vi "NI App Web Server.vi"() -> ()   [LabVIEW 2023]
uses:
  <vilib>/httpClient/POSTBuffer.vi
  Bad Idea Globals.vi
  <vilib>/httpClient/LabVIEWHTTPClient.lvlib
  <vilib>/Utility/TDMS File Viewer/NI_TDMS File Viewer.lvlib
panel:
  in  "Shutdown":bool
  in  "Freq":dbl=8.0
  in  "Phase":dbl
  in  "Amplitude":dbl=2.0
  out "Latest":waveform(dbl)(graph) caption="Latest Waveform from WebService"
  in  "Save":bool
  in  "Live":bool
  in  "Stop":bool
  in  "Start":bool
  out "WS_Shutdown":bool
  out "Running?":bool
  out "Commands":string[](array[string])
  out "Live":dynamicdata(graph) caption="Live Waveform (generated while \"Running\")"
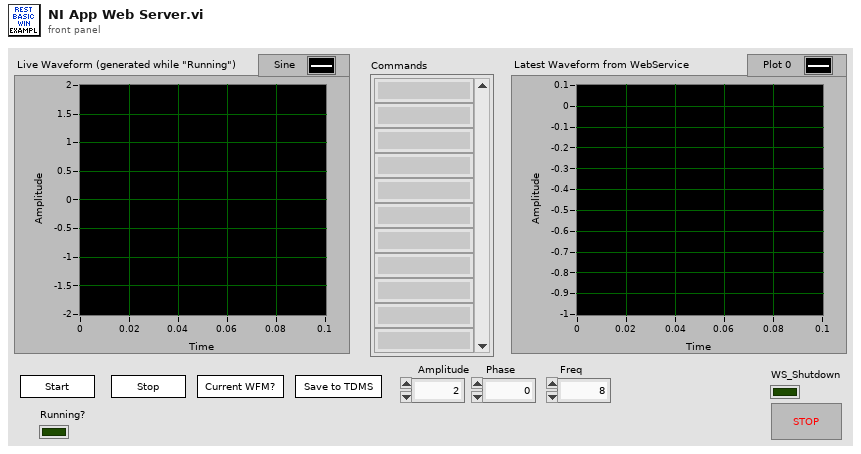
[diagram p1: front panel]
types:
  T1 = cluster{"Running":bool, "Amplitude":dbl, "Phase":dbl, "Freq":dbl}
  T2 = typedef "LabVIEWHTTPClient.lvlib/ClientHandle.ctl" = refnum<k1>
  T3 = enum16{"open", "open or create", "create or replace", "create", "open (read-only)"}
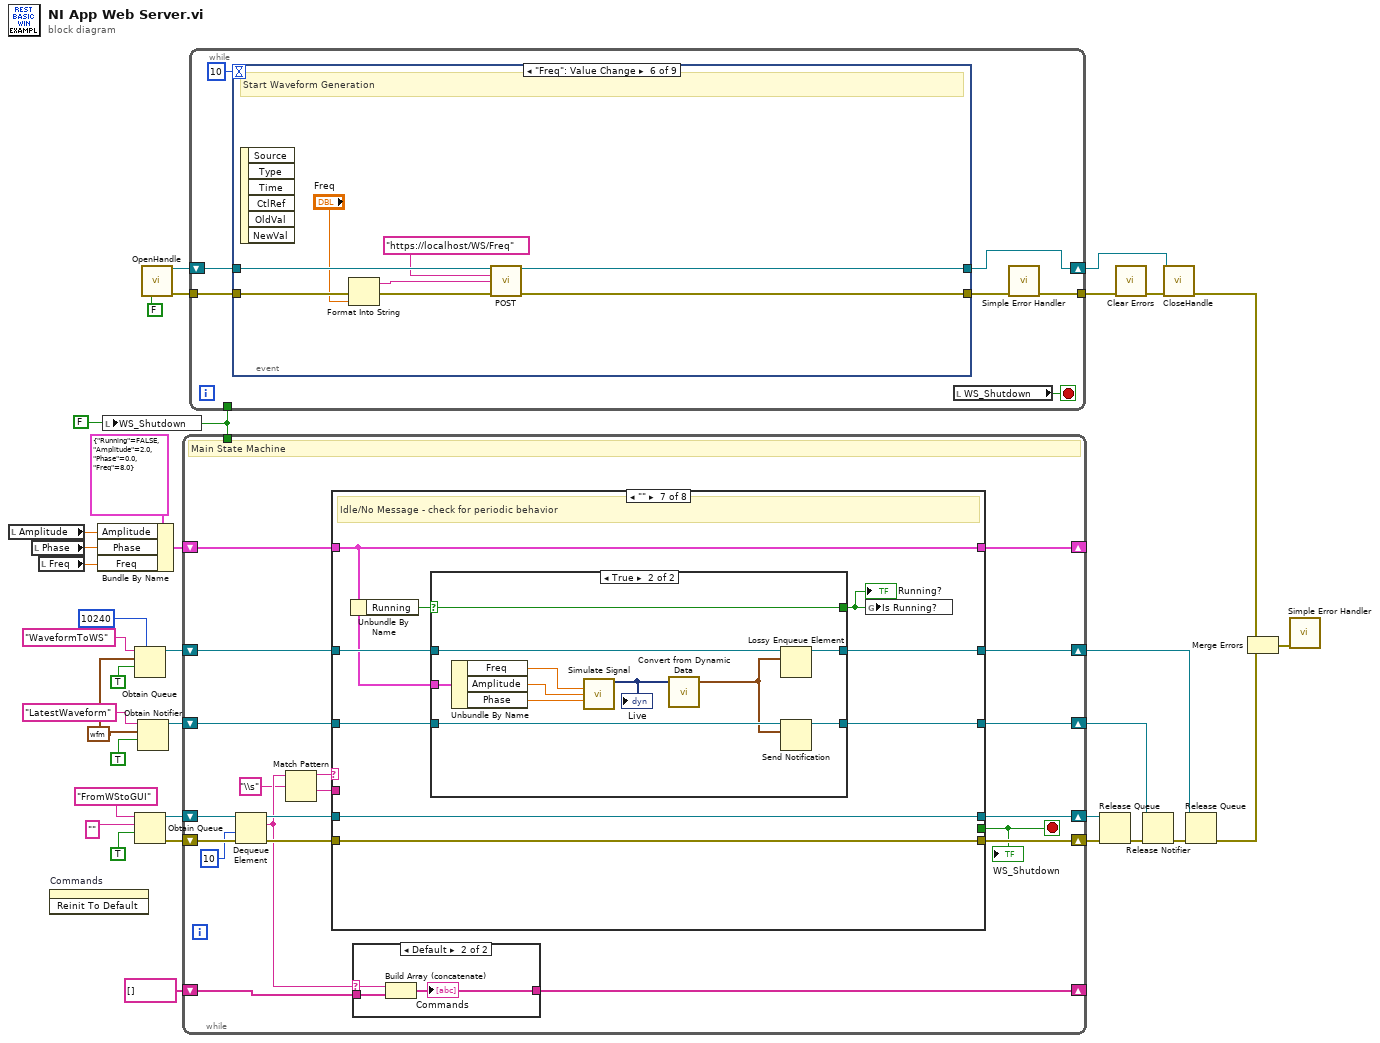
[diagram p0: block diagram]
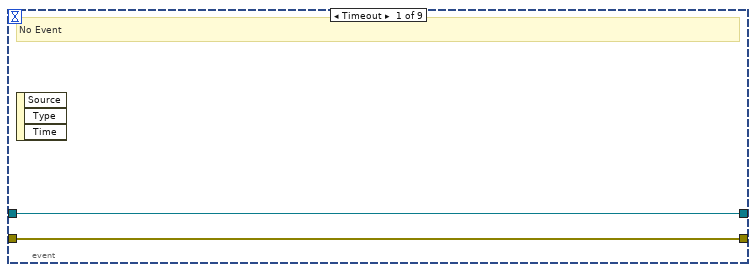
[diagram p2: hidden frame]
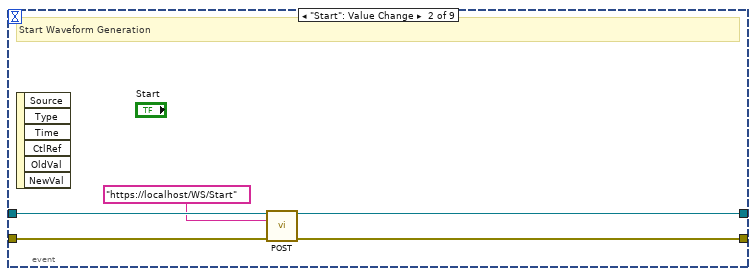
[diagram p3: hidden frame]
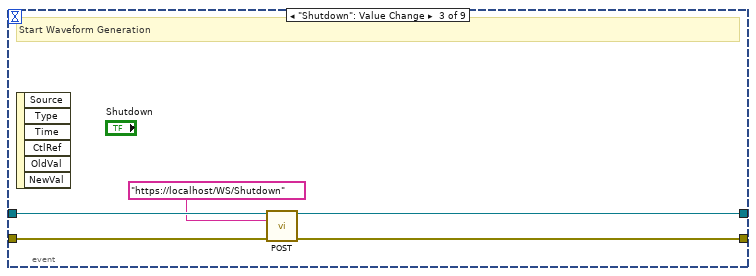
[diagram p4: hidden frame]
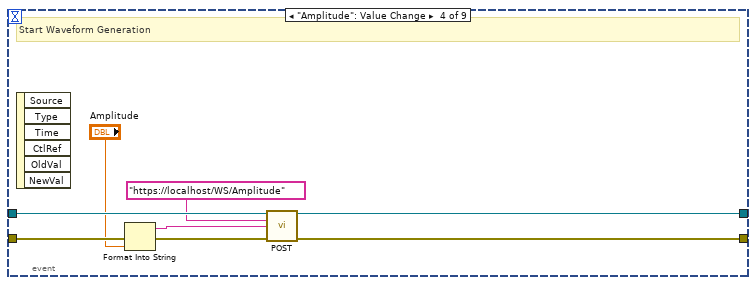
[diagram p5: hidden frame]
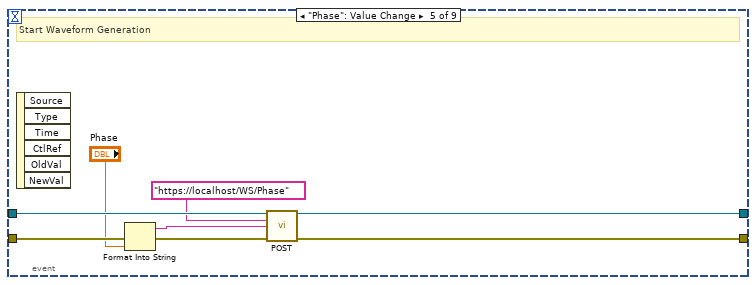
[diagram p6: hidden frame]
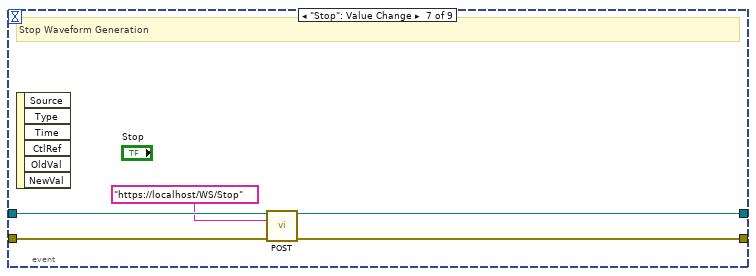
[diagram p7: hidden frame]
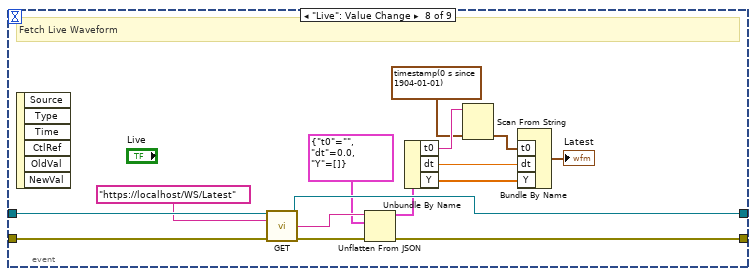
[diagram p8: hidden frame]
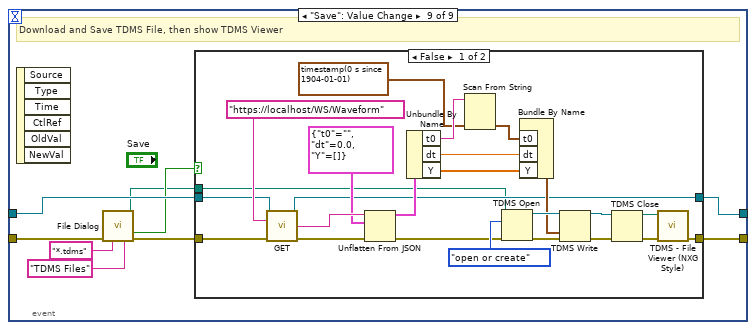
[diagram p9: hidden frame]
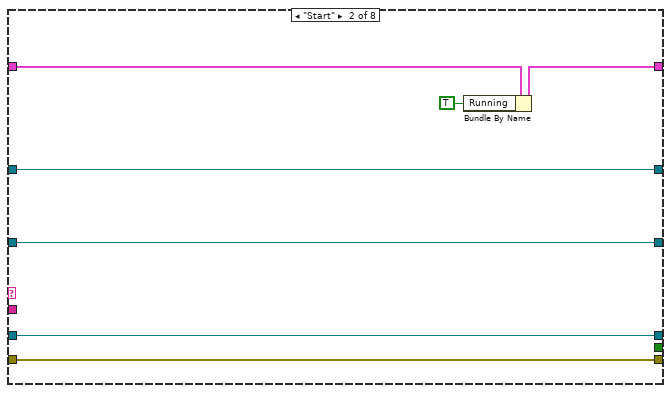
[diagram p13: hidden frame]
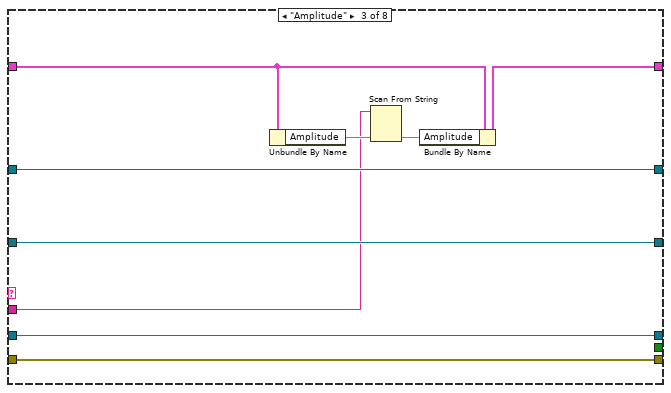
[diagram p14: hidden frame]
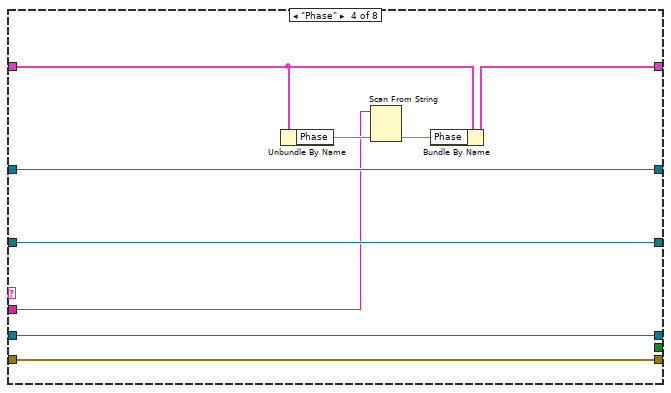
[diagram p15: hidden frame]
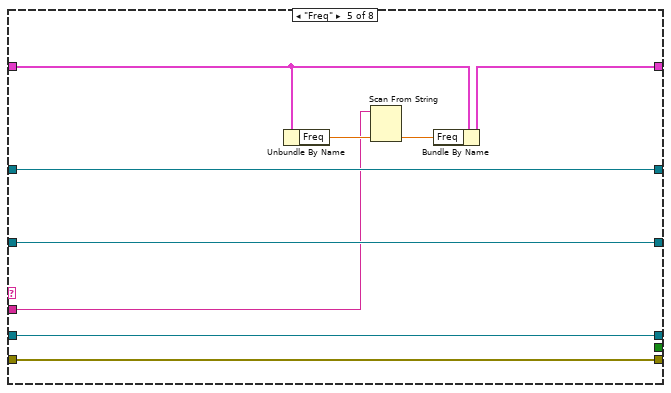
[diagram p16: hidden frame]
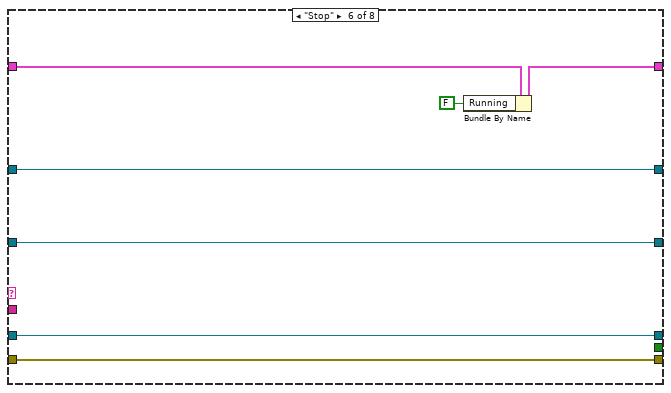
[diagram p17: hidden frame]
diagram:
  w15 = FALSE
  w28 = waveform(dbl) {"t0"=timestamp(0 s since 1904-01-01), "dt"=1.0, "Y"=[]}
  n1 = local read "Amplitude"() -> (w3:dbl)
  n2 = local read "Phase"() -> (w2:dbl)
  n3 = local read "Freq"() -> (w1:dbl)
  n4 = invoke on="Commands" class="Arr (strict)" method="Reinit To Default"() -> ()  [unwired: 3 in, 3 out]
  n5 = Bundle By Name(cluster=T1 {"Running"=FALSE, "Amplitude"=2.0, "Phase"=0.0, "Freq"=8.0}, "Amplitude"=w3, "Phase"=w2, "Freq"=w1) -> (w5:T1)
  n6 = local write "WS_Shutdown"(w15) -> ()
  n7 = Obtain Queue(max queue size (-1, unlimited)=10240, name (unnamed)="WaveformToWS", element data type=w28, create if not found? (T)=TRUE) -> (queue out=w27:refnum<queue>)  [unwired: 1 in, 2 out]
  n8 = Obtain Queue(name (unnamed)="FromWStoGUI", element data type="", create if not found? (T)=TRUE) -> (queue out=w32:refnum<queue>, error out=w33:errorcluster)  [unwired: 2 in, 1 out]
  n9 = Obtain Notifier(name (unnamed)="LatestWaveform", notification data type=w28, create if not found? (T)=TRUE) -> (notifier out=w29:refnum<notifier>)  [unwired: 1 in, 2 out]
  n10 = call <vilib>:"OpenHandle.vi"("verify server(true)"=FALSE) -> ("client handle out"=w19:T2, "error out"=w18:errorcluster)  [unwired: 13 in]
  n11 = while "Send to RT" {
    shift-right: [w49] -> w30
    shift-left: w33 -> [w55]
    shift-right: [w50] -> w31
    shift-left: w32 -> [w54]
    shift-right: [w47] -> w24
    shift-left: w29 -> [w48]
    shift-right: [w45] -> w23
    shift-left: w27 -> [w46]
    shift-right: [w43] -> _
    shift-left: w5 -> [w44]
    shift-right: [w41] -> _
    shift-left: string[] [] -> [w42]
    tunnel: w15 -> [_]
    stop <- w36 stop-if-true
    # "Main State Machine"
    n12 = Dequeue Element(queue=w54, timeout in ms (-1)=10, error in (no error)=w55) -> (queue out=w51:refnum<queue>, element=w40:string, error out=w52:errorcluster)  [unwired: 1 out]
    n13 = Match Pattern(string=w40, regular expression="\\s") -> (before substring=w39:string, after substring=w37:string)  [unwired: 1 in, 2 out]
    n14 = case shown="\"\"" w39 {
      tunnel: w52 -> [w63 w70 w79 w88 w97 w104 w113 w133]
      tunnel: w51 -> [w64 w71 w80 w89 w98 w105 w114 w134]
      tunnel: [w64 w71 w80 w89 w98 w105 w114 w134] -> w50
      tunnel: [w63 w70 w79 w88 w97 w104 w113 w133] -> w49
      tunnel: [_ _ _ _ _ _ _ TRUE] -> w36
      tunnel: w48 -> [w62 w69 w78 w87 w96 w103 w110 w131]
      tunnel: [w62 w69 w78 w87 w96 w103 w108 w131] -> w47
      tunnel: w46 -> [w61 w68 w77 w86 w95 w102 w111 w130]
      tunnel: [w61 w68 w77 w86 w95 w102 w109 w130] -> w45
      tunnel: w44 -> [w60 w65 w74 w83 w92 w99 w107 w129]
      tunnel: [w60 w66 w76 w85 w94 w100 w107 w129] -> w43
      tunnel: w37 -> [_ _ w72 w81 w90 _ _ _]
      frame Default {
      }
      frame "Start" {
        n15 = Bundle By Name(cluster=w65, "Running"=TRUE) -> (w66:T1)
      }
      frame "Amplitude" {
        n16 = Unbundle By Name(w74) -> ("Amplitude"=w73:dbl)
        n17 = Scan From String(input string=w72, default 1=w73) -> (output 1=w75:dbl)  [unwired: 3 in, 3 out]
        n18 = Bundle By Name(cluster=w74, "Amplitude"=w75) -> (w76:T1)
      }
      frame "Phase" {
        n19 = Unbundle By Name(w83) -> ("Phase"=w82:dbl)
        n20 = Scan From String(input string=w81, default 1=w82) -> (output 1=w84:dbl)  [unwired: 3 in, 3 out]
        n21 = Bundle By Name(cluster=w83, "Phase"=w84) -> (w85:T1)
      }
      frame "Freq" {
        n22 = Unbundle By Name(w92) -> ("Freq"=w91:dbl)
        n23 = Scan From String(input string=w90, default 1=w91) -> (output 1=w93:dbl)  [unwired: 3 in, 3 out]
        n24 = Bundle By Name(cluster=w92, "Freq"=w93) -> (w94:T1)
      }
      frame "Stop" {
        n25 = Bundle By Name(cluster=w99, "Running"=FALSE) -> (w100:T1)
      }
      frame "" {
        # "Idle/No Message - check for periodic behavior"
        n26 = Unbundle By Name(w107) -> ("Running"=w112:bool)
        n27 = case shown="True" w112 {
          selector: w112 -> [w115 w120]
          tunnel: w111 -> [w117 w122]
          tunnel: w110 -> [w116 w128]
          tunnel: [w117 w123] -> w109
          tunnel: [w116 w121] -> w108
          tunnel: w107 -> [_ w126]
          tunnel: [w115 w120] -> w106
          frame False {
          }
          frame True {
            n28 = Unbundle By Name(w126) -> ("Freq"=w127:dbl, "Amplitude"=w125:dbl, "Phase"=w124:dbl)
            n29 = call "Simulate Signal"("Frequency"=w127, "Amplitude"=w125, "Phase"=w124) -> ("Sine"=w119:dynamicdata)  [unwired: 11 in, 1 out]
            "Live" <- w119
            n30 = call "Convert from Dynamic Data"("Dynamic Data Type"=w119) -> ("Waveform"=w118:waveform(dbl))  [unwired: 3 in]
            n31 = Lossy Enqueue Element(queue=w122, element=w118) -> (queue out=w123:refnum<queue>)  [unwired: 1 in, 3 out]
            n32 = Send Notification(notification=w118, notifier=w128) -> (notifier out=w121:refnum<notifier>)  [unwired: 1 in, 1 out]
          }
        }
        "Running?" <- w106
        n33 = global write "Bad Idea Globals.vi" "Is Running?"(w106) -> ()
      }
      frame "Shutdown" {
      }
    }
    "WS_Shutdown" <- w36
    n34 = case shown="Default" w40 {
      selector: w40 -> [_ w59]
      tunnel: w42 -> [w56 w58]
      tunnel: [w56 w57] -> w41
      frame "\u0000" {
      }
      frame Default {
        n35 = Build Array (concatenate)(w59, w58) -> (w57:string[])
        "Commands" <- w57
      }
    }
  }
  n36 = while {
    shift-right: [w136] -> w7
    shift-left: w19 -> [w137]
    tunnel: w18 -> [w138]
    tunnel: [w135] -> w17
    tunnel: w15 -> [_]
    stop <- w141 stop-if-true
    n37 = event shown="[5] \"Freq\": Value Change" {
      selector: _ -> [_ _ _ _ _ _ _ _ _]
      dyn-events: _ -> [_ _ _ _ _ _ _ _ _]
      timeout: 10 -> [_ _ _ _ _ _ _ _ _]
      tunnel: [w142 w148 w153 w161 w169 w177 w182 w191 w203] -> w139
      tunnel: w138 -> [w142 w145 w150 w158 w166 w174 w179 w196 w201]
      tunnel: w137 -> [w143 w146 w151 w159 w167 w175 w180 w197 w204]
      tunnel: [w143 w147 w152 w160 w168 w176 w181 w192 w202] -> w136
      event Timeout {
        # "No Event"
        n38 = event-data() -> ()  [unwired: 1 in, 3 out]
      }
      event "Start": Value Change {
        # "Start Waveform Generation"
        n39 = event-data() -> ()  [unwired: 1 in, 6 out]
        n40 = call-poly <vilib>:"POST.vi"("client handle"=w146, "url"="https://localhost/WS/Start", "error in (no error)"=w145) -> ("client handle out"=w147:T2, "error out"=w148:errorcluster)  [unwired: 9 in, 2 out]
      }
      event "Shutdown": Value Change {
        # "Start Waveform Generation"
        n41 = event-data() -> ()  [unwired: 1 in, 6 out]
        n42 = call-poly <vilib>:"POST.vi"("client handle"=w151, "url"="https://localhost/WS/Shutdown", "error in (no error)"=w150) -> ("client handle out"=w152:T2, "error out"=w153:errorcluster)  [unwired: 9 in, 2 out]
      }
      event "Amplitude": Value Change {
        # "Start Waveform Generation"
        n43 = event-data() -> ()  [unwired: 1 in, 6 out]
        n44 = Format Into String(error in=w158, "Amplitude") -> (resulting string=w154:string, error out=w156:errorcluster)  [unwired: 2 in]
        n45 = call-poly <vilib>:"POST.vi"("client handle"=w159, "url"="https://localhost/WS/Amplitude", "buffer"=w154, "error in (no error)"=w156) -> ("client handle out"=w160:T2, "error out"=w161:errorcluster)  [unwired: 8 in, 2 out]
      }
      event "Phase": Value Change {
        # "Start Waveform Generation"
        n46 = event-data() -> ()  [unwired: 1 in, 6 out]
        n47 = Format Into String(error in=w166, "Phase") -> (resulting string=w163:string, error out=w164:errorcluster)  [unwired: 2 in]
        n48 = call-poly <vilib>:"POST.vi"("client handle"=w167, "url"="https://localhost/WS/Phase", "buffer"=w163, "error in (no error)"=w164) -> ("client handle out"=w168:T2, "error out"=w169:errorcluster)  [unwired: 8 in, 2 out]
      }
      event "Freq": Value Change {
        # "Start Waveform Generation"
        n49 = event-data() -> ()  [unwired: 1 in, 6 out]
        n50 = Format Into String(error in=w174, "Freq") -> (resulting string=w171:string, error out=w172:errorcluster)  [unwired: 2 in]
        n51 = call-poly <vilib>:"POST.vi"("client handle"=w175, "url"="https://localhost/WS/Freq", "buffer"=w171, "error in (no error)"=w172) -> ("client handle out"=w176:T2, "error out"=w177:errorcluster)  [unwired: 8 in, 2 out]
      }
      event "Stop": Value Change {
        # "Stop Waveform Generation"
        n52 = event-data() -> ()  [unwired: 1 in, 6 out]
        n53 = call-poly <vilib>:"POST.vi"("client handle"=w180, "url"="https://localhost/WS/Stop", "error in (no error)"=w179) -> ("client handle out"=w181:T2, "error out"=w182:errorcluster)  [unwired: 9 in, 2 out]
      }
      event "Live": Value Change {
        # "Fetch Live Waveform"
        n54 = event-data() -> ()  [unwired: 1 in, 6 out]
        n55 = call <vilib>:"GET.vi"("client handle"=w197, "url"="https://localhost/WS/Latest", "error in (no error)"=w196) -> ("client handle out"=w192:T2, "body"=w193:string, "error out"=w194:errorcluster)  [unwired: 9 in, 1 out]
        n56 = Unflatten From JSON(JSON string=w193, type and defaults=cluster{"t0":string, "dt":dbl, "Y":dbl[]} {"t0"="", "dt"=0.0, "Y"=[]}, error in (no error)=w194) -> (value=w188:cluster{"t0":string, "dt":dbl, "Y":dbl[]}, error out=w191:errorcluster)  [unwired: 4 in]
        n57 = Unbundle By Name(w188) -> ("t0"=w187:string, "dt"=w184:dbl, "Y"=w183:dbl[])
        n58 = Scan From String(input string=w187, default 1=timestamp(0 s since 1904-01-01)) -> (output 1=w185:timestamp)  [unwired: 3 in, 3 out]
        n59 = Bundle By Name("t0"=w185, "dt"=w184, "Y"=w183) -> (→"Latest":waveform(dbl))  [unwired: 1 in]
      }
      event "Save": Value Change {
        # "Download and Save TDMS File, then show TDMS Viewer"
        n60 = event-data() -> ()  [unwired: 1 in, 6 out]
        n61 = call "File Dialog"("error in"=w201, "pattern (all files)"="*.tdms", "pattern label"="TDMS Files") -> ("selected path"=w198:path, "cancelled"=w200:bool, "error out"=w199:errorcluster)  [unwired: 9 in, 1 out]
        n62 = case shown="False" w200 {
          tunnel: w204 -> [w216 w232]
          tunnel: [w208 w231] -> w203
          tunnel: [w213 w232] -> w202
          tunnel: w199 -> [w212 w231]
          tunnel: w198 -> [w211 _]
          frame False {
            n63 = call <vilib>:"GET.vi"("client handle"=w216, "url"="https://localhost/WS/Waveform", "error in (no error)"=w212) -> ("client handle out"=w213:T2, "body"=w228:string, "error out"=w229:errorcluster)  [unwired: 9 in, 1 out]
            n64 = Unflatten From JSON(JSON string=w228, type and defaults=cluster{"t0":string, "dt":dbl, "Y":dbl[]} {"t0"="", "dt"=0.0, "Y"=[]}, error in (no error)=w229) -> (value=w223:cluster{"t0":string, "dt":dbl, "Y":dbl[]}, error out=w210:errorcluster)  [unwired: 4 in]
            n65 = Unbundle By Name(w223) -> ("t0"=w226:string, "dt"=w222:dbl, "Y"=w221:dbl[])
            n66 = Scan From String(input string=w226, default 1=timestamp(0 s since 1904-01-01)) -> (output 1=w224:timestamp)  [unwired: 3 in, 3 out]
            n67 = TDMS Open(8:w210, 10:T3."open or create" ("operation (0:open)"), 11:w211) -> (0:w219:errorcluster, 3:w218:refnum<k34>)  [unwired: 4 in]
            n68 = Bundle By Name("t0"=w224, "dt"=w222, "Y"=w221) -> (w215:waveform(dbl))  [unwired: 1 in]
            n69 = TDMS Write(0:w218, 9:w215, 11:w219) -> (4:w214:refnum<k34>, 15:w220:errorcluster)  [unwired: 3 in, 2 out]
            n70 = TDMS Close(8:w220, 11:w214) -> (0:w209:errorcluster, 3:w207:path)
            n71 = call <vilib>:"TDMS - File Viewer (NXG Style).vi"("error in"=w209, "file in"=w207) -> ("error out"=w208:errorcluster)  [unwired: 8 in, 1 out]
          }
          frame True {
          }
        }
      }
    }
    n72 = local read "WS_Shutdown"() -> (w141:bool)
    n73 = call <vilib>:"Simple Error Handler.vi"("error in (no error)"=w139) -> ("error out"=w135:errorcluster)  [unwired: 4 in, 4 out]
  }
  n74 = Release Queue(queue=w31, error in (no error)=w30) -> (error out=w26:errorcluster)  [unwired: 1 in, 2 out]
  n75 = call <vilib>:"Clear Errors.vi"("error in (no error)"=w17) -> ("error out"=w6:errorcluster)  [unwired: 5 in, 1 out]
  n76 = Release Notifier(notifier=w24, error in (no error)=w26) -> (error out=w25:errorcluster)  [unwired: 1 in, 2 out]
  n77 = call <vilib>:"CloseHandle.vi"("client handle"=w7, "error in (no error)"=w6) -> ("error out"=w9:errorcluster)  [unwired: 13 in]
  n78 = Release Queue(queue=w23, error in (no error)=w25) -> (error out=w10:errorcluster)  [unwired: 1 in, 2 out]
  n79 = Merge Errors(w9, w10) -> (w8:errorcluster)
  n80 = call <vilib>:"Simple Error Handler.vi"("error in (no error)"=w8) -> ()  [unwired: 4 in, 5 out]
